vi "GE5565 Disable DMA Interrupt (Cluster) mod.vi"(4 "error in (no error)":errorcluster, 7 "VMIC reference in":T1) -> (0 "error out":errorcluster, 3 "VMIC reference out":T1)   [LabVIEW 2019, in "GE_RM_Real Time.lvlib"]
uses:
  GE_RM_Real Time.lvlib
  Select Event Type.ctl
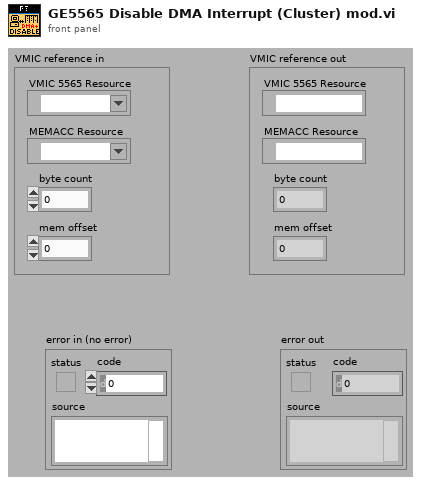
[diagram p1: front panel]
types:
  T1 = cluster{"VMIC 5565 Resource":refnum<visa-resource-name>, "MEMACC Resource":refnum<visa-resource-name>, "byte count":u32, "mem offset":u32}
  T2 = typedef "Select Event Type.ctl" = u32
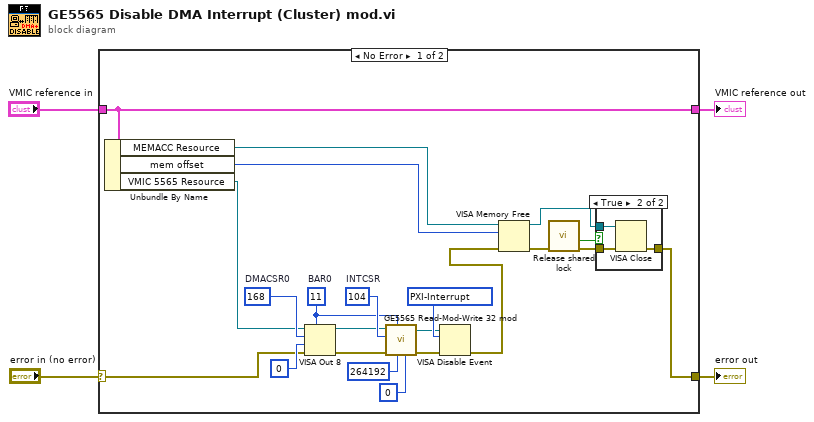
[diagram p0: block diagram]
diagram:
  n1 = case shown="No Error" "error in (no error)" {
    selector: "error in (no error)" -> [w24 w31]
    tunnel: "VMIC reference in" -> [w9 w32]
    tunnel: [w9 w32] -> w1
    tunnel: [w23 w31] -> w3
    frame No Error {
      w17 = u16 11  # BAR0
      w16 = T2 1073684514 items=["ServiceRequest"=1073684491, "Trigger"=3221168138, "Clear"=1073684493, "VXI-Signal"=1073684512, "VXI/VME-Interrupt"=3221168161, "VXI/VME-Sysfail"=1073684509, "VXI/VME-Sysreset"=1073684510, "GPIB-CIC"=1073684498, "GPIB-Talk"=1073684499, "GPIB-Listen"=1073684500, "PXI-Interrupt"=1073684514, "AllEnabled"=1073709055] ("Event Type")
      w22 = u32 104  # INTCSR
      w26 = u32 168  # DMACSR0
      n2 = Unbundle By Name(w9) -> ("MEMACC Resource"=w11:refnum<visa-resource-name>, "mem offset"=w12:u32, "VMIC 5565 Resource"=w13:refnum<visa-resource-name>)
      n3 = VISA Out 8(7:w17, 8:w24, 9:u8 0 ("value (0)"), 10:w26, 11:w13) -> (0:w18:errorcluster, 3:w19:refnum<visa-resource-name>)
      n4 = call "GE5565 Read-Mod-Write 32 mod.vi"("value"=u32 0, "inv bit mask"=u32 264192 ("value"), "address space (13: BAR2)"=w17, "error in (no error)"=w18, "offset (0)"=w22, "VISA resource name"=w19) -> ("error out"=w14:errorcluster, "VISA resource name out"=w15:refnum<visa-resource-name>)  [unwired: 4 in]
      n5 = VISA Disable Event(8:w14, 10:w16, 11:w15) -> (0:w10:errorcluster)  [unwired: 1 in, 1 out]
      n6 = VISA Memory Free(8:w10, 10:w12, 11:w11) -> (0:w8:errorcluster, 3:w6:refnum<visa-resource-name>)
      n7 = call "Release shared lock.vi"("error in (no error)"=w8) -> ("error out"=w7:errorcluster, "Safe to delete"=w5:bool)  [unwired: 9 in]
      n8 = case shown="True" w5 {
        tunnel: [w27 w30] -> w23
        tunnel: w7 -> [w27 w29]
        tunnel: w6 -> [_ w28]
        frame False {
        }
        frame True {
          n9 = VISA Close(VISA resource name=w28, error in (no error)=w29) -> (error out=w30:errorcluster)
        }
      }
    }
    frame Error {
    }
  }
  "error out" <- w3
  "VMIC reference out" <- w1
